vi "TTLToggle.vi"() -> ()   [LabVIEW 2011]
doc: "This sample project is built upon the standard state machine template and shows how you could create an application that acquires, analyzes, and presents data. It includes functionality for presenting configuration dialogs, preserving settings between executions, loading and saving data, as well as exporting graph images and text files.\n\nIt is most appropriate for data that is acquired instantly as it does not allow for screen updates mid acquisition nor does it allow for continuous streaming to disk."
panel:
  in  "Toggle\nTTL 2":bool
  in  "Toggle\nTTL 1":bool
  out "Toggle Status":dbl
  out "USB_Open Status":dbl
  in  "Stop":bool
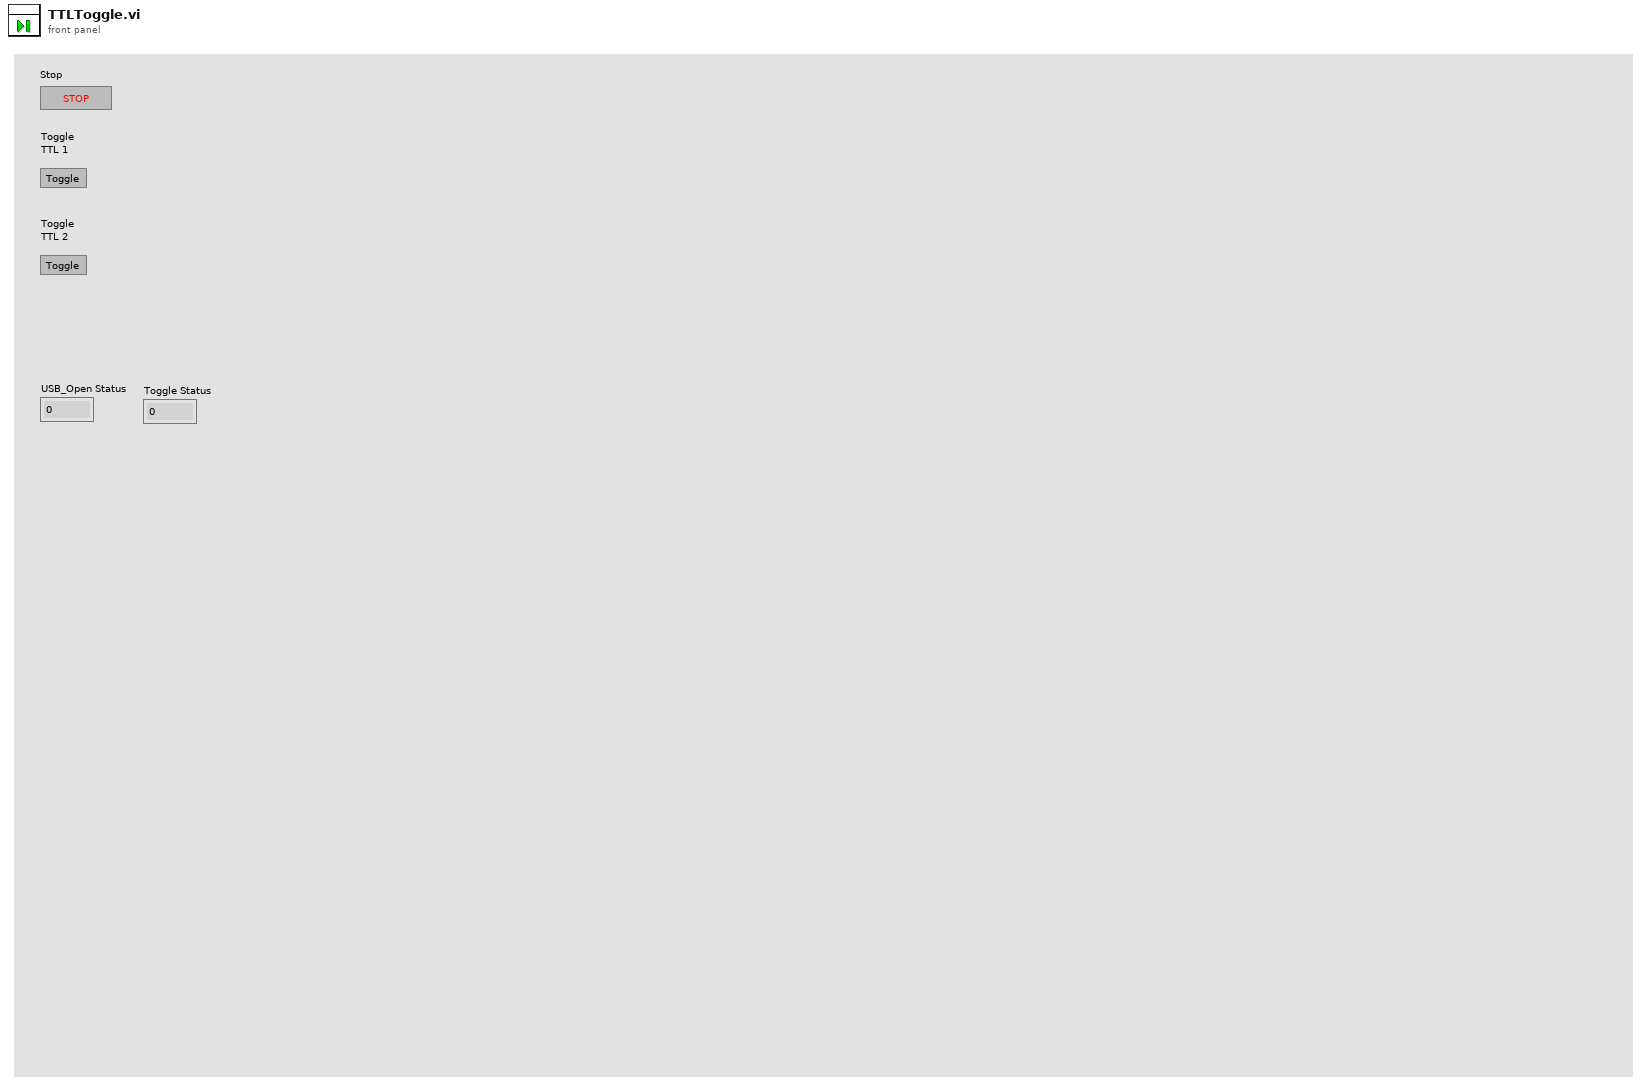
[diagram p1: front panel]
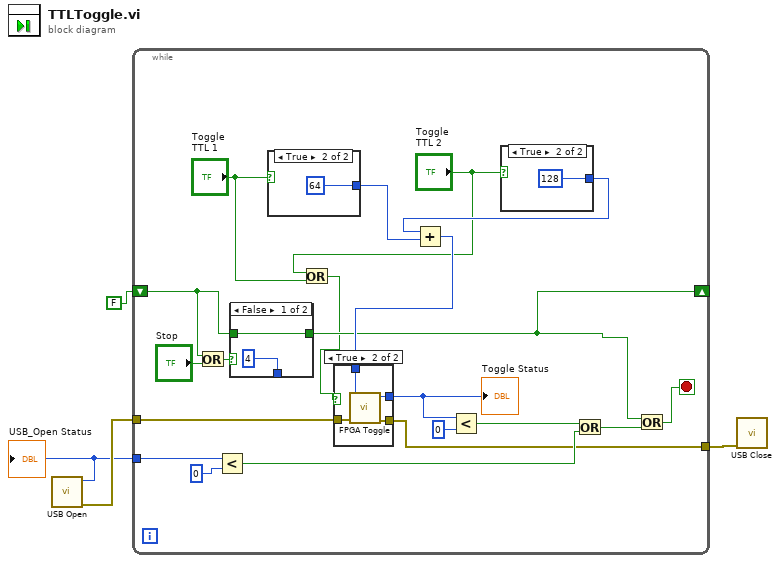
[diagram p0: block diagram]
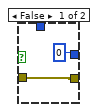
[diagram p2: hidden frame]
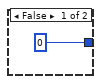
[diagram p3: hidden frame]
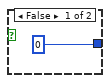
[diagram p4: hidden frame]
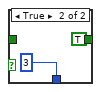
[diagram p5: hidden frame]
diagram:
  n1 = call "USB Open.vi"() -> ("error out"=w4:errorcluster, "function return"=w2:i32)  [unwired: 10 in]
  "USB_Open Status" <- w2
  n2 = while {
    tunnel: w4 -> [w14]
    tunnel: [w13] -> w3
    tunnel: w2 -> [w21]
    shift-right: [w8] -> _
    shift-left: FALSE -> [w15]
    stop <- w23 stop-if-true
    n3 = Or(x=w15, y="Stop") -> (x .or. y?=w17:bool)
    n4 = Less?(x=w21, y=0) -> (x < y?=w19:bool)
    n5 = case shown="False" w17 {
      tunnel: [4 3] -> _
      tunnel: [w36 TRUE] -> w8
      tunnel: w15 -> [w36 _]
      frame False {
      }
      frame True {
      }
    }
    n6 = case shown="True" "Toggle\nTTL 1" {
      tunnel: [0 64] -> w10
      frame False {
      }
      frame True {
      }
    }
    n7 = Or(x="Toggle\nTTL 2", y="Toggle\nTTL 1") -> (x .or. y?=w7:bool)
    n8 = case shown="True" "Toggle\nTTL 2" {
      tunnel: [0 128] -> w11
      frame False {
      }
      frame True {
      }
    }
    n9 = Add(x=w11, y=w10) -> (x+y=w9:i32)
    n10 = case shown="True" w7 {
      tunnel: w14 -> [w26 w30]
      tunnel: [w26 w29] -> w13
      tunnel: [0 w28] -> w12
      tunnel: w9 -> [_ w27]
      frame False {
      }
      frame True {
        n11 = call "FPGA Toggle.vi"("error in (no error)"=w30, "fpgaCommand"=w27) -> ("error out"=w29:errorcluster, "function return"=w28:i32)  [unwired: 8 in]
      }
    }
    "Toggle Status" <- w12
    n12 = Less?(x=w12, y=0) -> (x < y?=w20:bool)
    n13 = Or(x=w20, y=w19) -> (x .or. y?=w18:bool)
    n14 = Or(x=w8, y=w18) -> (x .or. y?=w23:bool)
  }
  n15 = call "USB Close.vi"("error in (no error)"=w3) -> ()  [unwired: 9 in, 2 out]
